vi "Controller.vi"(10 "Controller":refnum<class "Controller.lvclass">, 11 "Processing In":refnum<class "Processing.lvclass">) -> (0 "error out":errorcluster, 3 "Processing":refnum<class "Processing.lvclass">)   [LabVIEW 2020, in "HTTP Server.lvlib" / "Server.lvclass"]
uses:
  Server.lvclass
  Server.lvclass/Server.ctl
  Session/Session.lvclass
  Processing Step.ctl
  HTTP Server.lvlib
  Processing/Processing.lvclass
  Controller/Controller.lvclass
  C:/dev/lv20CE/relink/lv-http-server/HTTP Server/Controller/Controller.lvclass
  C:/dev/lv20CE/relink/lv-http-server/HTTP Server/Handler/Handler.lvclass
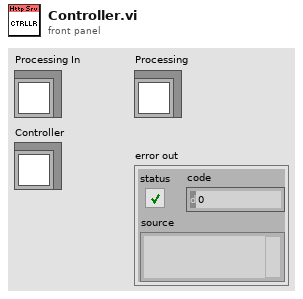
[diagram p1: front panel]
types:
  T1 = typedef "HTTP Server.lvlib/Processing Step.ctl" = enum16{"Connection", "Request", "Routing", "Controller Init", "Controller", "Response", "Complete", "Exception"}
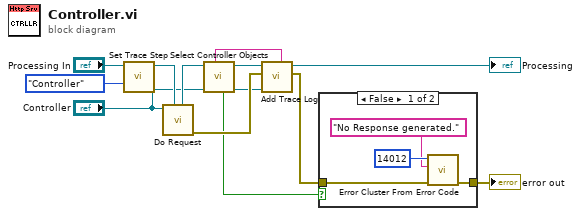
[diagram p0: block diagram]
diagram:
  n1 = call "Set Trace Step.vi"("Processing Step"=Processing_Step."Controller", "Processing in"="Processing In") -> ("Processing out"=w2:refnum<class "Processing.lvclass">)  [unwired: 9 in]
  n2 = call-dynamic "Do Request.vi"("Processing In"=w2, "Controller in"="Controller") -> ("error out"=w12:errorcluster, "Processing"=w6:refnum<class "Processing.lvclass">)  [unwired: 8 in]
  n3 = call "Select Controller Objects.vi"("Processing In"=w6) -> ("Processing"=w7:refnum<class "Processing.lvclass">, "Response?"=w10:bool, "Trace Message"=w8:string)  [unwired: 8 in]
  n4 = call "Add Trace Log.vi"("Info"=w8, "LabVIEW Object"="Controller", "error in (no error)"=w12, "Processing in"=w7) -> ("error out"=w4:errorcluster, "Processing out"=→"Processing":refnum<class "Processing.lvclass">)  [unwired: 6 in]
  n5 = case shown="False" w10 {
    tunnel: [w16 w17] -> w11
    tunnel: w4 -> [w13 w17]
    frame False {
      n6 = call <vilib>:"Error Cluster From Error Code.vi"("error in (no error)"=w13, "error message (\"\")"="No Response generated." ("format string"), "error code (0)"=14012) -> ("error out"=w16:errorcluster)  [unwired: 6 in]
    }
    frame True {
    }
  }
  "error out" <- w11
